vi "ROI group interface.vi"(6 "Demo (F)":bool, 7 "New group (F)":bool, 10 "POI group info cluster in":T1 {"Group region specifier cluster"."Contours"."Type" items=["No Selection", "Point", "Line", "Rectangle", "Oval", "Polygon", "Freehand Region", "Annulus", "Unused2", "Unused3", "Broken Line", "Freehand Line", "Rotated Rectangle"]}) -> (1 "POI group info cluster":T1 {"Group region specifier cluster"."Contours"."Type" items=["No Selection", "Point", "Line", "Rectangle", "Oval", "Polygon", "Freehand Region", "Annulus", "Unused2", "Unused3", "Broken Line", "Freehand Line", "Rotated Rectangle"]}, 2 "Cancelled":bool, 3 "Image ref out":T3)   [LabVIEW 2017]
uses:
  <vilib>/vision/Image Controls.llb/IMAQ Image.ctl
  ROI group info cluster.ctl
  Typedefs/Get-Set-Clear Control.ctl
  Global variables/gl_Functional Imaging-Global variables.vi
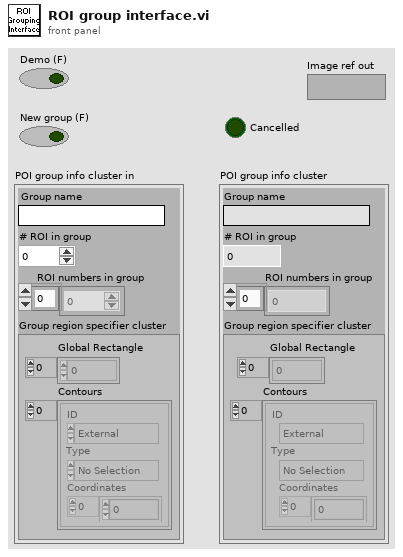
[diagram p1: front panel]
types:
  T1 = typedef "ROI group info cluster.ctl" = cluster{"Group name":string, "# ROI in group":i32, "ROI numbers in group":i32[], "Group region specifier cluster":T2}
  T2 = typedef "ROI Descriptor" = cluster{"Global Rectangle":i32[], "Contours":cluster{"ID":enum32{"External", "Internal"}, "Type":u32, "Coordinates":i32[]}[]}
  T3 = typedef "IMAQ Image.ctl" = refnum<image>
  T4 = typedef "Get-Set-Clear Control.ctl" = enum16{"Get", "Set", "Clear"}
  T5 = typedef "ROI parameters data type.ctl" = cluster{"ROI index":dbl, "ROI ID":dbl, "ROI Time (ns)":dbl, "Pixels in ROI":dbl, "X start":dbl, "Y start":dbl, "Z start":dbl, "X stop":dbl, "Y stop":dbl, "Z stop":dbl, "Angle (deg)":dbl, "Composite ID":dbl, "Number of lines":dbl, "Frame Size":dbl, "Zoom":dbl, "Laser Power (%)":dbl, "ROI group ID":dbl}
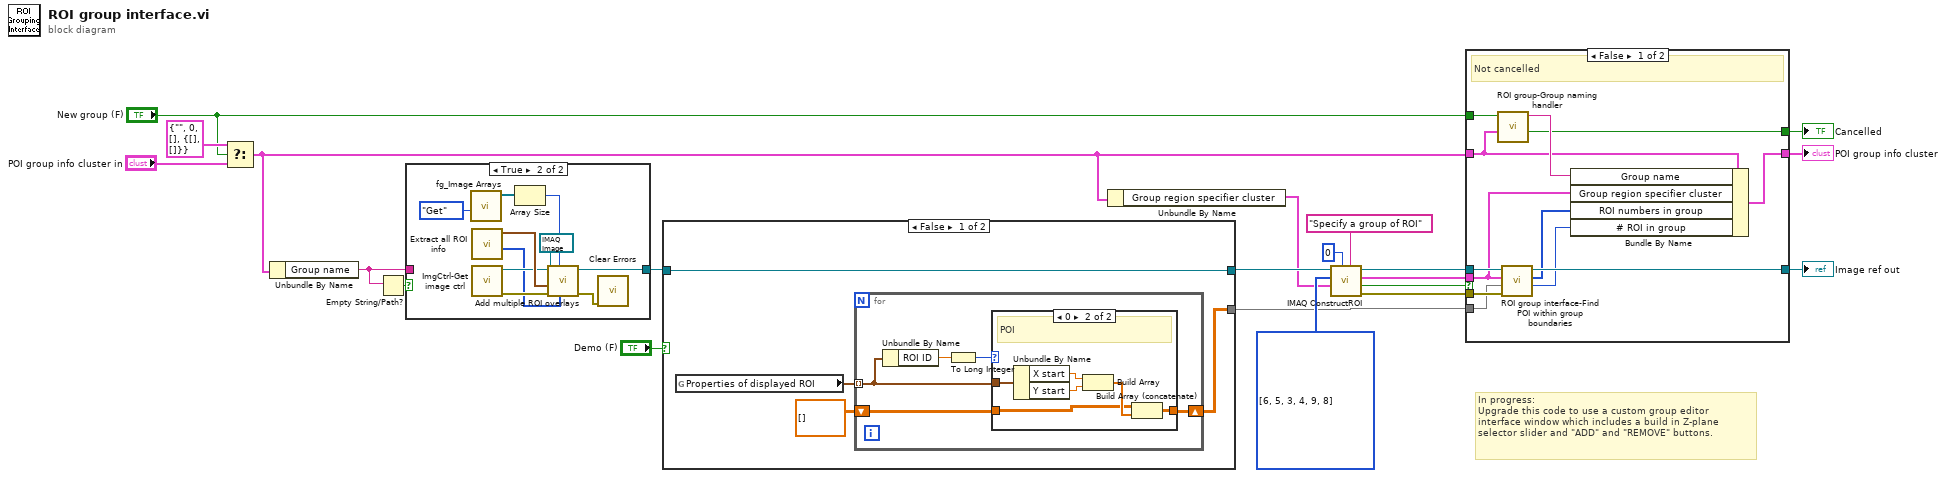
[diagram p0: block diagram]
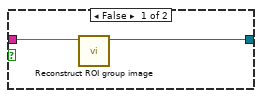
[diagram p2: hidden frame]
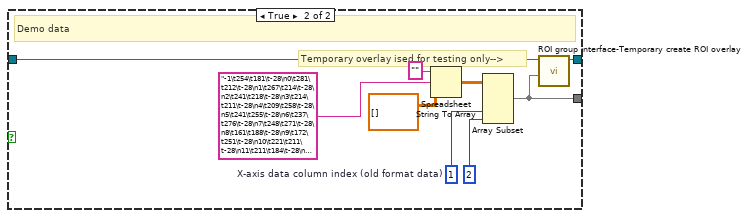
[diagram p4: hidden frame]
diagram:
  w19 = u32[] [6, 5, 3, 4, 9, 8] items=["No Selection", "Point", "Line", "Rectangle", "Oval", "Polygon", "Freehand Region", "Annulus", "Zoom", "Pan", "Broken Line", "Freehand Line", "Rotated Rectangle"] ("Tools")
  # "In progress:\nUpgrade this code to use a custom group editor interface window which includes a build in Z-plane selector slider and \"ADD\" and \"REMOVE\" buttons."
  n1 = Select(t=T1 {"Group name"="", "# ROI in group"=0, "ROI numbers in group"=[], "Group region specifier cluster"={"Global Rectangle"=[], "Contours"=[]}} ("POI group info cluster in"), s="New group (F)", f="POI group info cluster in") -> (s? t:f=w3:T1)
  n2 = Unbundle By Name(w3) -> ("Group name"=w1:string)
  n3 = Empty String/Path?(string/path=w1) -> (empty?=w2:bool)
  n4 = case shown="True" w2 {
    tunnel: [w23 w31] -> w5
    tunnel: w1 -> [w22 _]
    frame False {
      n5 = call "Reconstruct ROI group image.vi"("Name of ROI group to search for"=w22) -> ("Image to display"=w23:T3)  [unwired: 8 in, 2 out]
    }
    frame True {
      n6 = call "fg_Image Arrays.vi"("Function"=Get-Set-Clear_Control."Get") -> ("Red Images Array"=w27:T3[])  [unwired: 9 in, 1 out]
      n7 = call "Extract all ROI info.vi"() -> ("Zero-based index of the Z-plane the indexed ROI belongs to"=w28:i32[], "[ROI info]"=w33:T5[])  [unwired: 10 in]
      n8 = call "ImgCtrl-Get image ctrl.vi"() -> ("error out"=w30:errorcluster, "Image"=w32:T3)  [unwired: 10 in]
      n9 = Array Size(array=w27) -> (size(s)=w25:i32)
      n10 = call "Add multiple ROI overlays.vi"("[ROI index] (unity based)"=w28, "# of Z-planes"=w25, "error in"=w30, "[ROI info]"=w33, "Image 2 in"=T3 refnum, "Image 1 in"=w32) -> ("error out"=w24:errorcluster, "Image 1 out"=w31:T3)  [unwired: 3 in, 1 out]
      n11 = call <vilib>:"Clear Errors.vi"("error in (no error)"=w24) -> ()  [unwired: 5 in, 2 out]
    }
  }
  n12 = case shown="False" "Demo (F)" {
    tunnel: [w37 w58] -> w16
    tunnel: [w34 w57] -> w15
    tunnel: w5 -> [w37 w56]
    frame False {
      n13 = global read "gl_Functional Imaging-Global variables.vi" "Properties of displayed ROI"() -> (w35:T5[])
      n14 = for {
        tunnel: w35 -> [w41] mode=indexing
        shift-right: [w40] -> w34
        shift-left: dbl[][] [] -> [w39]
        n15 = Unbundle By Name(w41) -> ("ROI ID"=w42:dbl)
        n16 = To Long Integer(number=w42) -> (32bit integer=w38:i32)
        n17 = case shown="0" w38 {
          tunnel: w41 -> [_ w49]
          tunnel: [w43 w45] -> w40
          tunnel: w39 -> [w43 w44]
          frame Default {
          }
          frame 0 {
            # "POI"
            n18 = Unbundle By Name(w49) -> ("X start"=w48:dbl, "Y start"=w47:dbl)
            n19 = Build Array(w48, w47) -> (w46:dbl[])
            n20 = Build Array (concatenate)(w44, w46) -> (w45:dbl[][])
          }
        }
      }
    }
    frame True {
      w55 = 1  # X-axis data column index (old format data)
      # "Temporary overlay ised for testing only-->"
      # "Demo data"
      n21 = Spreadsheet String To Array(format string="", spreadsheet string="-1\t254\t181\t-28\n0\t281\t212\t-28\n1\t267\t214\t-28\n2\t241\t218\t-28\n3\t214\t211\t-28\n4\t209\t258\t-28\n5\t241\t255\t-28\n6\t237\t276\t-28\n7\t248\t271\t-28\n8\t161\t188\t-28\n9\t172\t251\t-28\n10\t221\t211\t-28\n11\t211\t184\t-28\n12\t264\t175\t-28\n13\t264\t201\t-28\n14\t232\t209\t-28\n15\t202\t171\t-28\n16\t184\t161\t-28\n17\t99\t124\t-28\n18\t71\t225\t-28\n19\t185\t340\t-28\n20\t343\t106\t-28\n21\t250\t206\t-22\n22\t249\t220\t-22\n23\t217\t216\t-22\n24\t181\t223\t-22\n25\t255\t235\t-22\n26\t274\t235\t-22\n27\t352\t305\t-22\n28\t301\t292\t-22\n29\t278\t75\t-22\n30\t405\t204\t-22\n31\t323\t417\t-22\n32\t320\t211\t-16\n33\t239\t217\t-16\n34\t212\t182\t-16\n35\t180\t234\t-16\n36\t221\t295\t-16\n37\t281\t301\t-16\n38\t277\t233\t-16\n39\t240\t203\t-16\n40\t223\t259\t-16\n41\t175\t196\t-16\n42\t166\t190\t-16\n43\t156\t229\t-16\n44\t302\t220\t-16\n45\t271\t126\t-16\n46\t257\t109\t-16\n47\t213\t90\t-16\n48\t116\t77\t-16\n49\t459\t416\t-16\n50\t239\t246\t-10\n51\t272\t258\t-10\n52\t253\t187\t-10\n53\t234\t159\t-10\n54\t192\t156\t-10\n55\t166\t182\t-10\n56\t131\t213\t-10\n57\t148\t239\t-10\n58\t160\t299\t-10\n59\t210\t350\t-10\n60\t340\t347\t-10\n61\t369\t300\t-10\n62\t323\t182\t-10\n63\t280\t149\t-10\n64\t221\t136\t-10\n65\t385\t84\t-10\n66\t382\t341\t-10\n67\t306\t105\t-10\n68\t256\t210\t-4\n69\t194\t245\t-4\n70\t274\t312\t-4\n71\t268\t255\t-4\n72\t189\t226\t-4\n73\t193\t183\t-4\n74\t200\t126\t-4\n75\t304\t150\t-4\n76\t336\t167\t-4\n77\t369\t212\t-4\n78\t364\t263\t-4\n79\t119\t234\t-4\n80\t131\t299\t-4\n81\t183\t348\t-4\n82\t301\t365\t-4\n83\t249\t258\t-4\n84\t239\t202\t2\n85\t202\t256\t2\n86\t284\t289\t2\n87\t312\t236\t2\n88\t275\t182\t2\n89\t205\t113\t2\n90\t152\t147\t2\n91\t126\t229\t2\n92\t153\t364\t2\n93\t229\t371\t2\n94\t362\t356\t2\n95\t357\t211\t2\n96\t365\t169\t2\n97\t302\t55\t2\n98\t178\t54\t2\n99\t60\t139\t2\n100\t237\t218\t8\n101\t264\t286\t8\n102\t277\t223\t8\n103\t225\t261\t8\n104\t152\t129\t8\n105\t373\t346\t8\n106\t370\t146\t8\n107\t107\t240\t8\n108\t239\t146\t14\n109\t243\t84\t14\n110\t243\t69\t14\n111\t308\t394\t14\n112\t120\t331\t14\n113\t72\t215\t14\n114\t280\t193\t20\n115\t257\t245\t20\n116\t204\t193\t20\n117\t418\t137\t20\n118\t429\t210\t20\n119\t193\t233\t26\n120\t190\t94\t26\n121\t406\t317\t26\n122\t251\t187\t-22\n123\t234\t148\t-22\n124\t264\t204\t-28\n125\t436\t168\t-28\n126\t261\t237\t-4\n", array type (2D Dbl)=dbl[][] []) -> (array=w51:dbl[][])  [unwired: 1 in]
      n22 = Array Subset(array=w51, index (col)=w55, length (col)=2 ("length")) -> (w57:dbl[][])  [unwired: 2 in]
      n23 = call "ROI group interface-Temporary create ROI overlay.vi"("ROI X-Y data"=w57, "Image In"=w56) -> ("Image Out"=w58:T3)  [unwired: 8 in, 1 out]
    }
  }
  n24 = Unbundle By Name(w3) -> ("Group region specifier cluster"=w9:T2)
  n25 = call "IMAQ ConstructROI"("Prompt"="Specify a group of ROI", "Window Number (-1...15)"=0, "ROI Descriptor In (None)"=w9, "Tools"=w19, "Image"=w16) -> ("error out"=w20:errorcluster, "Cancel"=w10:bool, "ROI Descriptor Out"=w13:T2, "Image Out (duplicate)"=w14:T3)  [unwired: 3 in]
  n26 = case shown="False" w10 {
    selector: w10 -> [_ w71]
    tunnel: w14 -> [w70 w73]
    tunnel: w20 -> [w69 _]
    tunnel: w13 -> [w62 _]
    tunnel: w15 -> [w68 _]
    tunnel: w3 -> [w61 w72]
    tunnel: [w67 w73] -> w18
    tunnel: [w65 w72] -> w12
    tunnel: "New group (F)" -> [w60 _]
    tunnel: [w59 w71] -> w6
    frame False {
      # "Not cancelled"
      n27 = call "ROI group-Group naming handler.vi"("POI group info cluster in"=w61, "New group (F)"=w60) -> ("Cancelled?"=w59:bool, "Group name"=w63:string)  [unwired: 8 in]
      n28 = call "ROI group interface-Find POI within group boundaries.vi"("error in (no error)"=w69, "X-Y coordinates array of POI"=w68, "ROI Descriptor Out"=w62, "Image ref in"=w70) -> ("# of POI in group"=w66:i32, "ROI to be grouped"=w64:i32[], "Image ref shift out"=w67:T3)  [unwired: 4 in, 1 out]
      n29 = Bundle By Name(cluster=w61, "Group name"=w63, "Group region specifier cluster"=w62, "ROI numbers in group"=w64, "# ROI in group"=w66) -> (w65:T1)
    }
    frame True {
      # "Cancelled"
    }
  }
  "Image ref out" <- w18
  "POI group info cluster" <- w12
  "Cancelled" <- w6
